vi "Text Get Section Info.vi"(8 "Error In":errorcluster, 10 "Rows Where Whitespace Starts":i32[](array[numeric]), 11 "Receipt Lines":string[](array[string])) -> (0 "Error Out":errorcluster, 1 "Footer Info":T1, 2 "Main Body Info":T1, 3 "Header Info":T1)   [LabVIEW 2018, in "Receipt Parsing.lvlib"]
uses:
  Receipt Parsing.lvlib
  Section Info--cluster.ctl
  Action.ctl
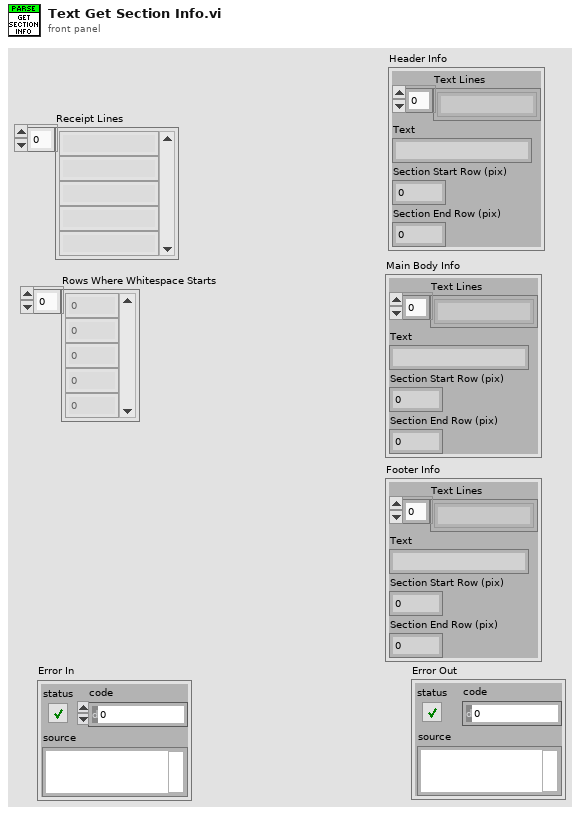
[diagram p1: front panel]
types:
  T1 = typedef "Receipt Parsing.lvlib/Section Info--cluster.ctl" = cluster{"Text Lines":string[], "Text":string, "Section Start Row (pix)":i32, "Section End Row (pix)":i32}
  T2 = cluster{"Header Info":T1, "Main Body Info":T1, "Footer Info":T1}
  T3 = typedef "Receipt Parsing.lvlib/Action.ctl" = enum16{"Init", "Read Image Text", "Text Get Sections", "Sections Get Data", "Close"}
  T4 = cluster{"Receipt Lines":string[], "Rows Where Whitespace Starts":i32[]}
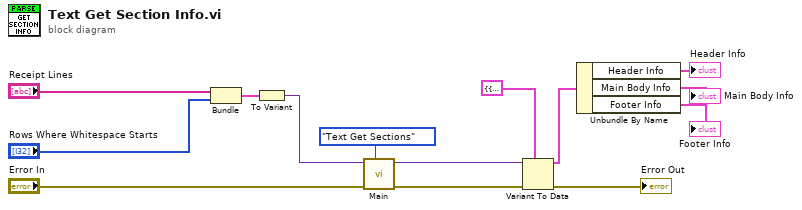
[diagram p0: block diagram]
diagram:
  n1 = Bundle("Receipt Lines"="Receipt Lines", "Rows Where Whitespace Starts"="Rows Where Whitespace Starts") -> (w10:T4)  [unwired: 1 in]
  n2 = To Variant(anything=w10) -> (Variant=w12:variant)
  n3 = call "Main.vi"("Action"=Action."Text Get Sections", "Error In"="Error In", "Data In"=w12) -> ("Error Out"=w6:errorcluster, "Data Out"=w5:variant)  [unwired: 7 in]
  n4 = Variant To Data(error in=w6, type=T2 {"Header Info"={"Text Lines"=[], "Text"="", "Section Start Row (pix)"=0, "Section End Row (pix)"=0}, "Main Body Info"={"Text Lines"=[], "Text"="", "Section Start Row (pix)"=0, "Section End Row (pix)"=0}, "Footer Info"={"Text Lines"=[], "Text"="", "Section Start Row (pix)"=0, "Section End Row (pix)"=0}} ("Section Data out"), Variant=w5) -> (data=w4:T2, error out=→"Error Out":errorcluster)
  n5 = Unbundle By Name(w4) -> ("Header Info"=→"Header Info":T1, "Main Body Info"=→"Main Body Info":T1, "Footer Info"=→"Footer Info":T1)
